vi "File.Move_Copy Files from Dir to Dir, Overwrite if Exists.vi"(6 "SkipIfExists(F)/Overwrite(T)":bool=TRUE, 7 "Move(F)/Copy(T)":bool=TRUE, 8 "error in":errorcluster, 9 "File Name Pattern":string, 10 "Dest Dir":path, 11 "Source Dir":path) -> (0 "error out":errorcluster, 3 "Count":i32)   [LabVIEW 2018]
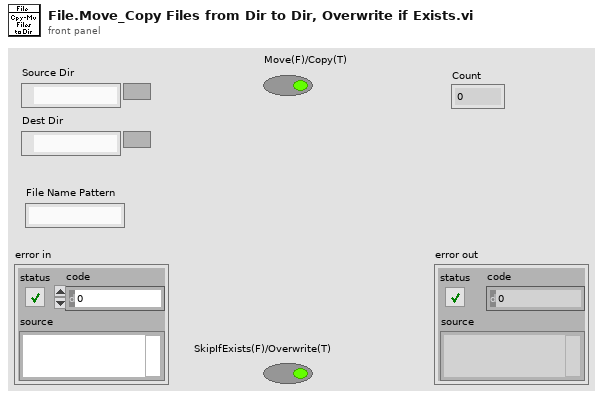
[diagram p1: front panel]
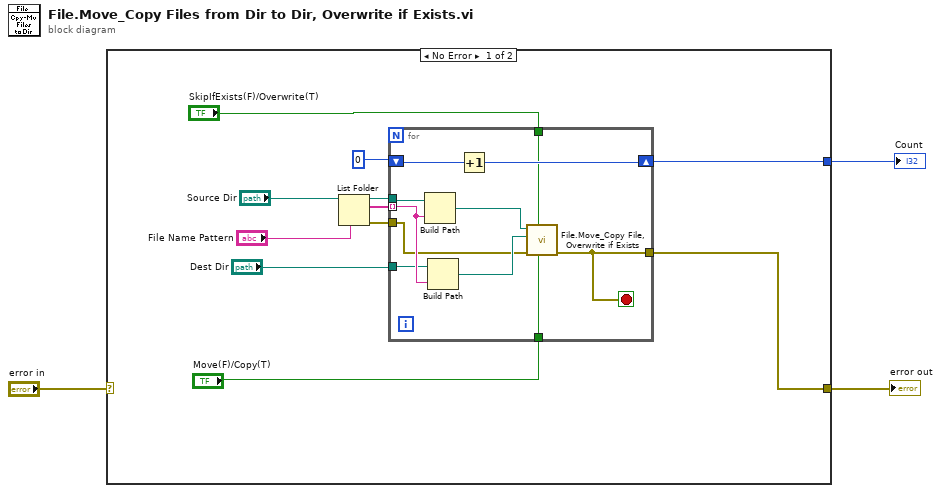
[diagram p0: block diagram]
diagram:
  n1 = case shown="No Error" "error in" {
    selector: "error in" -> [_ w26]
    tunnel: [w9 w26] -> w3
    tunnel: [w7 _] -> w2
    frame No Error {
      n2 = List Folder(path="Source Dir", pattern="File Name Pattern") -> (path out=w14:path, filenames=w13:string[], error out=w4:errorcluster)  [unwired: 2 in, 1 out]
      n3 = for {
        tunnel: w14 -> [w25]
        tunnel: w13 -> [w24] mode=indexing
        tunnel: "Dest Dir" -> [w23]
        tunnel: [w20] -> w9
        shift-right: [w18] -> w7
        shift-left: 0 -> [w19]
        tunnel: "Move(F)/Copy(T)" -> [w17]
        tunnel: "SkipIfExists(F)/Overwrite(T)" -> [w16]
        tunnel: w4 -> [w15]
        stop <- w20 stop-if-true
        n4 = Build Path(base path=w25, name or relative path=w24) -> (appended path=w22:path)
        n5 = Build Path(base path=w23, name or relative path=w24) -> (appended path=w21:path)
        n6 = Increment(x=w19) -> (x+1=w18:i32)
        n7 = call "File.Move_Copy File, Overwrite if Exists.vi"("Move(F)/Copy(T)"=w17, "SkipIfExists(F)/Overwrite(T)"=w16, "error in"=w15, "Target Path"=w21, "Source Path"=w22) -> ("error out"=w20:errorcluster)  [unwired: 5 in, 1 out]
      }
    }
    frame Error {
    }
  }
  "Count" <- w2
  "error out" <- w3
